vi "Drive Immediate.vi"(6 "Command Info In":T1, 7 "Description":string, 8 "Deadband Value":dbl=0.01, 9 "Spin Setpoint":dbl, 10 "Y Setpoint":dbl, 11 "X Setpoint":dbl) -> (0 "Command Info Out":T1)   [LabVIEW 2016]
doc: "Often used for joystick control, this VI checks to see that the joystick axes are outside the deadband and updates the motors appropriately."
uses:
  <vilib>/Rock Robotics/WPI/Framework/Command Status Info.ctl
  <vilib>/Rock Robotics/WPI/Framework/Completion Status.ctl
  <vilib>/Rock Robotics/WPI/Framework/Completion Notifier.ctl
  Implementation/Drive Setpoints.ctl
  Implementation/Drive Operations.ctl
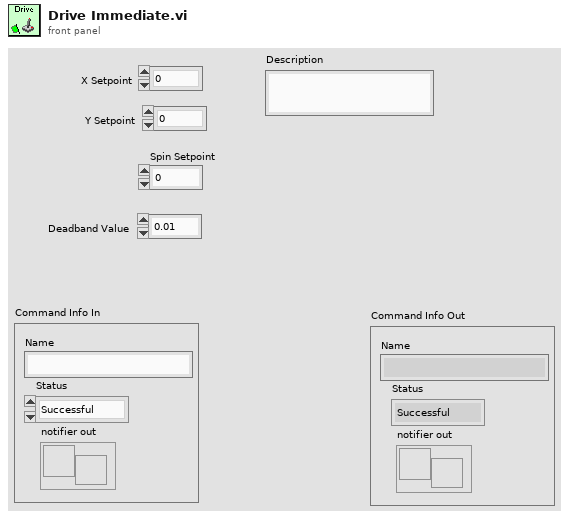
[diagram p1: front panel]
types:
  T1 = typedef "Command Status Info.ctl" = cluster{"Name":string, "Status":T2, "notifier out":T3}
  T2 = typedef "Completion Status.ctl" = enum16{"Successful", "Aborted", "Incomplete"}
  T3 = typedef "Completion Notifier.ctl" = refnum<notifier>
  T4 = typedef "Drive Setpoints.ctl" = cluster{"Operation":T5, "X Setpoint":dbl, "Y Setpoint":dbl, "Duration":dbl, "Twist Setpoint":dbl}
  T5 = typedef "Drive Operations.ctl" = enum16{"Reserve", "Read Current", "Immediate", "Drive for Time", "Drive for Distance"}
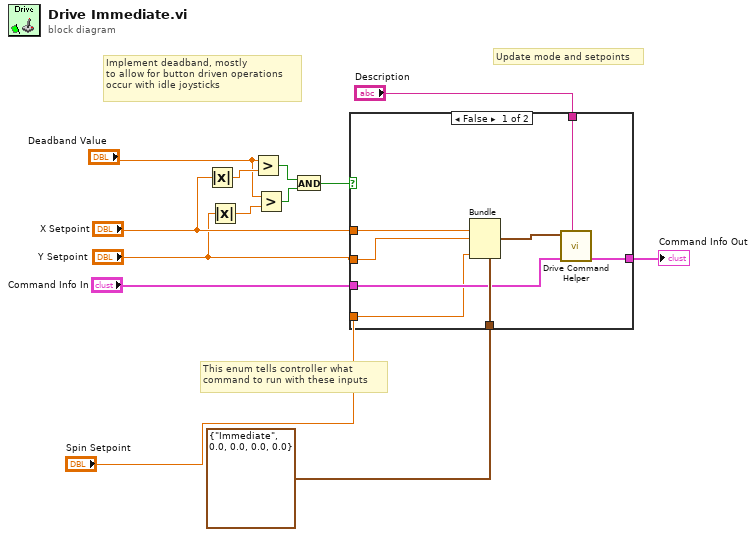
[diagram p0: block diagram]
diagram:
  # "This enum tells controller what \ncommand to run with these inputs"
  # "Implement deadband, mostly\nto allow for button driven operations\noccur with idle joysticks"
  # "Update mode and setpoints"
  n1 = Absolute Value(x="X Setpoint") -> (abs(x)=w13:dbl)
  n2 = Absolute Value(x="Y Setpoint") -> (abs(x)=w5:dbl)
  n3 = Greater?(x="Deadband Value", y=w13) -> (0:w7:bool)
  n4 = Greater?(x="Deadband Value", y=w5) -> (0:w3:bool)
  n5 = And(x=w7, y=w3) -> (x .and. y?=w6:bool)
  n6 = case shown="False" w6 {
    tunnel: "X Setpoint" -> [w21 _]
    tunnel: T4 {"Operation"=enum."Immediate", "X Setpoint"=0.0, "Y Setpoint"=0.0, "Duration"=0.0, "Twist Setpoint"=0.0} ("SubSystem Data") -> [w20 _]
    tunnel: [w19 w22] -> w12
    tunnel: "Command Info In" -> [w18 w22]
    tunnel: "Description" -> [w16 _]
    tunnel: "Y Setpoint" -> [w15 _]
    tunnel: "Spin Setpoint" -> [w14 _]
    frame False {
      n7 = Bundle(cluster=w20, "X Setpoint"=w21, "Y Setpoint"=w15, "Twist Setpoint"=w14) -> (w17:T4)  [unwired: 2 in]
      n8 = call "Drive Command Helper.vi"("Description"=w16, "Command Info In"=w18, "SubSystem Data"=w17) -> ("Command Info Out"=w19:T1)  [unwired: 7 in, 1 out]
    }
    frame True {
    }
  }
  "Command Info Out" <- w12
